vi "Localize_Particles-9-2.vi"(4 "Keep Nega-\ntive Values?":bool, 5 "# channel":u8, 6 "error IN":errorcluster, 7 "[IN] Filtering Settings":T1, 8 "[IN] Destination Image":T2, 9 "[IN] Frame":T2) -> (0 "error OUT":errorcluster, 2 "Histogram Graph":T3 {"Incremental Value" format="%.2f"; "Starting Value" format="%.2f"}, 3 "[OUT] LoG Processed Image":T2)   [LabVIEW 2013]
uses:
  <vilib>/vision/Image Controls.llb/IMAQ Image.ctl
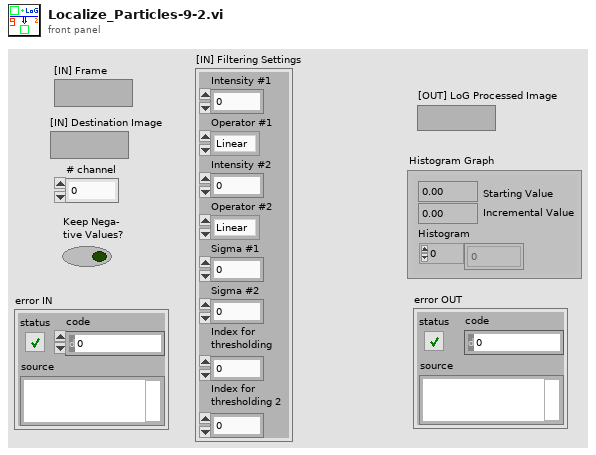
[diagram p1: front panel]
types:
  T1 = cluster{"Intensity #1":sgl, "Operator #1":enum32{"Linear", "Log", "Exp", "Square", "Square root", "Power X", "Power 1/X"}, "Intensity #2":sgl, "Operator #2":enum32{"Linear", "Log", "Exp", "Square", "Square root", "Power X", "Power 1/X"}, "Sigma #1":dbl, "Sigma #2":dbl, "Index for \nthresholding":u8, "Index for \nthresholding 2":u8}
  T2 = typedef "IMAQ Image.ctl" = refnum<image>
  T3 = cluster{"Starting Value":sgl, "Incremental Value":sgl, "Histogram":u32[]}
  T4 = enum32{"Linear", "Log", "Exp", "Square", "Square root", "Power X", "Power 1/X"}
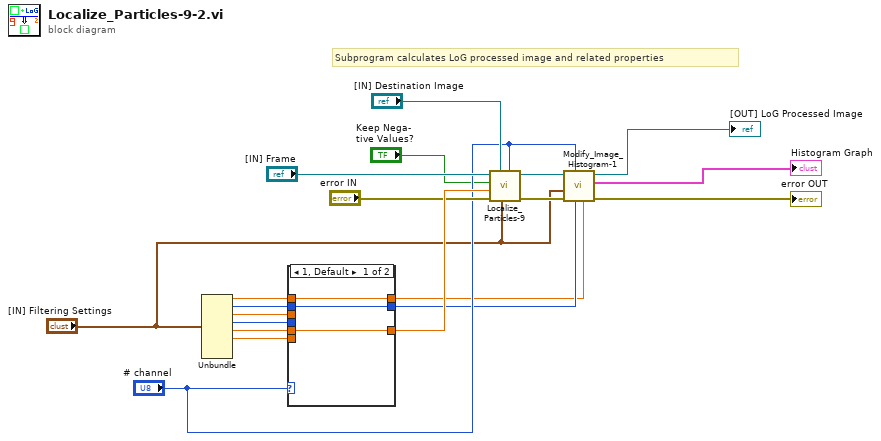
[diagram p0: block diagram]
diagram:
  # "Subprogram calculates LoG processed image and related properties"
  n1 = Unbundle("[IN] Filtering Settings") -> ("Intensity #1"=w20:sgl, "Operator #1"=w19:T4, "Intensity #2"=w18:sgl, "Operator #2"=w17:T4, "Sigma #1"=w16:dbl, "Sigma #2"=w15:dbl)  [unwired: 2 out]
  n2 = case shown="1, Default" "# channel" {
    tunnel: w20 -> [w23 _]
    tunnel: w19 -> [w22 _]
    tunnel: [w23 w26] -> w3
    tunnel: [w22 w25] -> w4
    tunnel: w18 -> [_ w26]
    tunnel: w17 -> [_ w25]
    tunnel: w16 -> [w21 _]
    tunnel: w15 -> [_ w24]
    tunnel: [w21 w24] -> w11
    frame 1, Default {
    }
    frame 2 {
    }
  }
  n3 = call "Localize_Particles-9.vi"("# channel"="# channel", "[IN] Filtering Settings"="[IN] Filtering Settings", "[IN] Destination Image"="[IN] Destination Image", "error IN"="error IN", "[IN] Sigma"=w11, "Keep Nega-\ntive Values?"="Keep Nega-\ntive Values?", "[IN] Frame"="[IN] Frame") -> ("error OUT"=w14:errorcluster, "[OUT] LoG Processed Image"=w13:T2)  [unwired: 1 in, 1 out]
  n4 = call "Modify_Image_Histogram-1.vi"("[IN] Parameter"=w3, "[IN] Operator"=w4, "# channel"="# channel", "error IN"=w14, "[IN] Filtering Settings"="[IN] Filtering Settings", "[IN] LoG Processed Image"=w13) -> ("error OUT"=→"error OUT":errorcluster, "[OUT] Histogram"=→"Histogram Graph":T3, "[OUT] Histogram Modified Image"=→"[OUT] LoG Processed Image":T2)  [unwired: 2 in, 1 out]
